vi "SP_BreakDown_Manage1.vi"() -> ()   [LabVIEW 2017]
uses:
  <vilib>/addons/database/Connection.llb/DB Tools Open Connec (Path).vi
  Globle/Login Data.vi
  <vilib>/addons/database/NI_Database_API.lvlib
panel:
  in  "Cancel Button - Archive":bool
  out "Stakeholder":string
  out "Role Id":string
  in  "Download 2":bool
  in  "Get Rport 2":bool
  in  "Manage 2":bool
  out "Table 2":string[][](array[string])
  out "error out":errorcluster
  in  "error in (no error)":errorcluster
  out "Table":string[][](table)
  in  "Shift":string(combo)
  in  "Station":string(combo)
  in  "To Date":timestamp format="%<%Y-%m-%d>T"
  in  "From Date":timestamp format="%<%Y-%m-%d>T"
  in  "Stakeholder":string(combo)
  # "Breakdown Manage"
  # "Designed And Developed By - Infinity Automation Systems Pvt. Ltd."
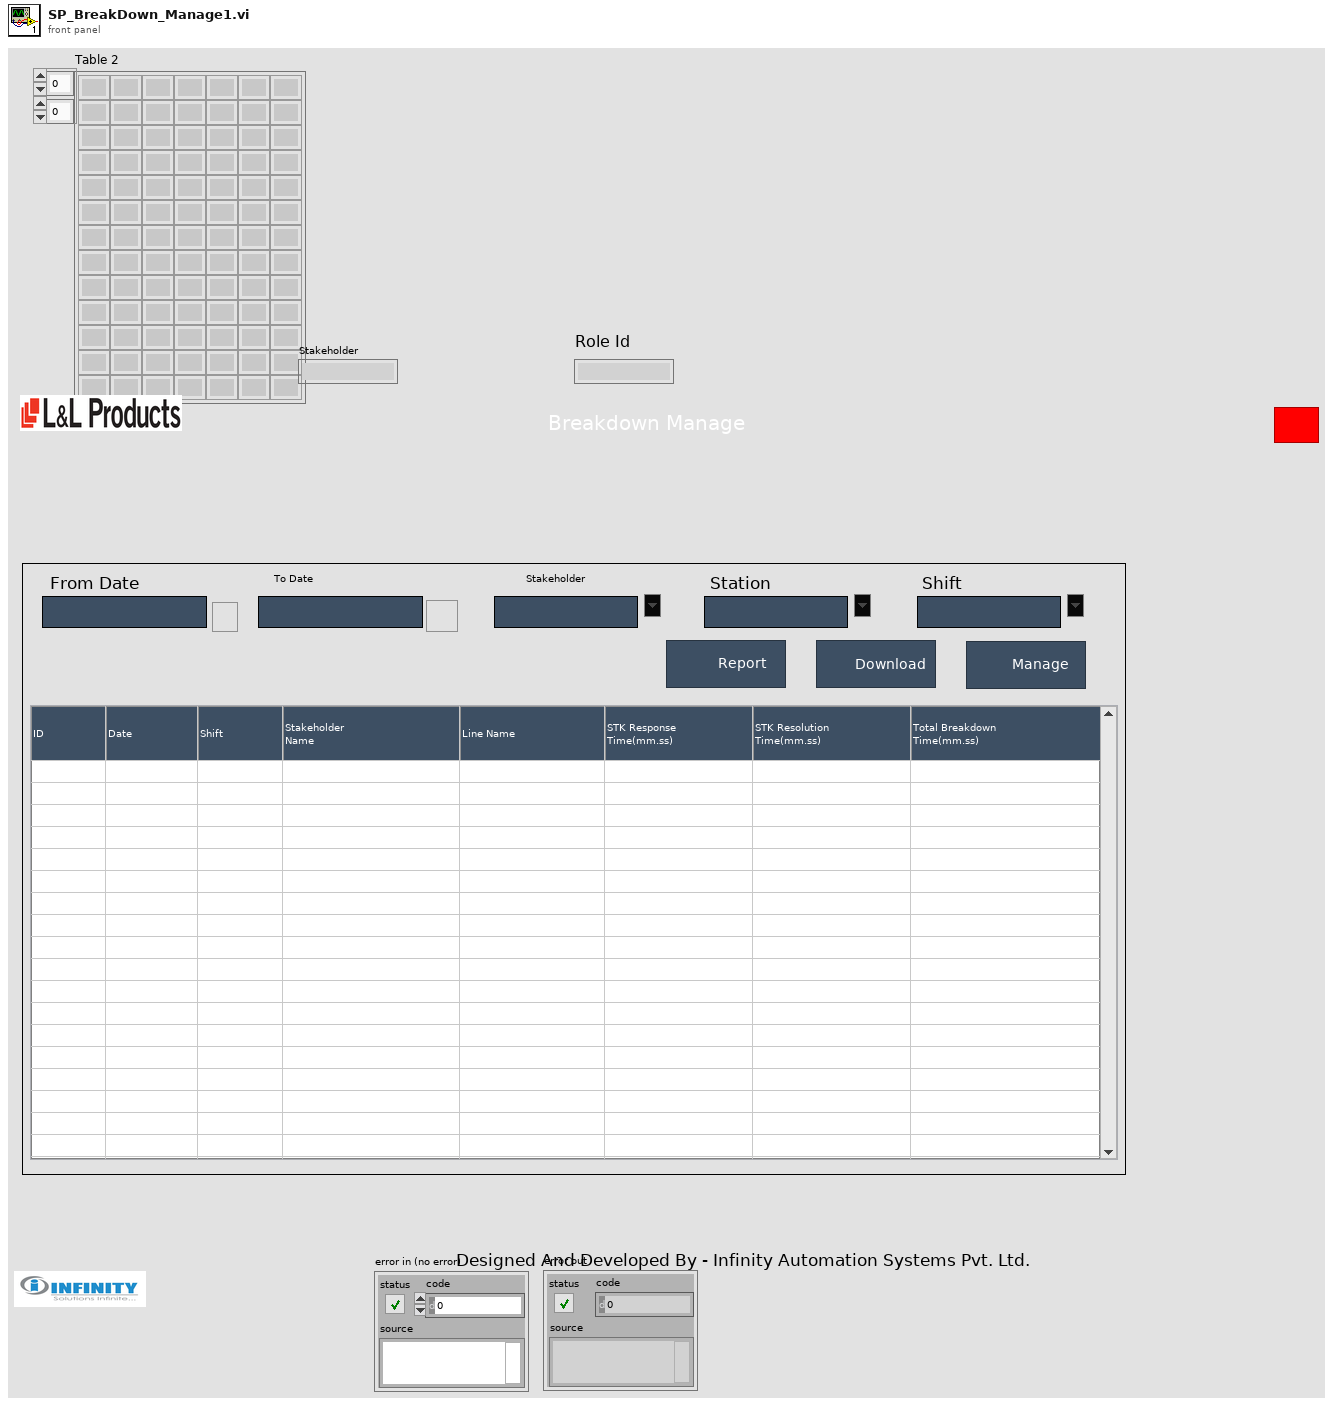
[diagram p1: front panel]
types:
  T1 = typedef "NI_Database_API.lvlib/Conn ObjectReference.ctl" = refnum<k1>
  T2 = enum32{"invalid app kind", "Development System", "Run Time System", "Student Edition", "Embedded LabVIEW", "Evaluation", "Custom"}
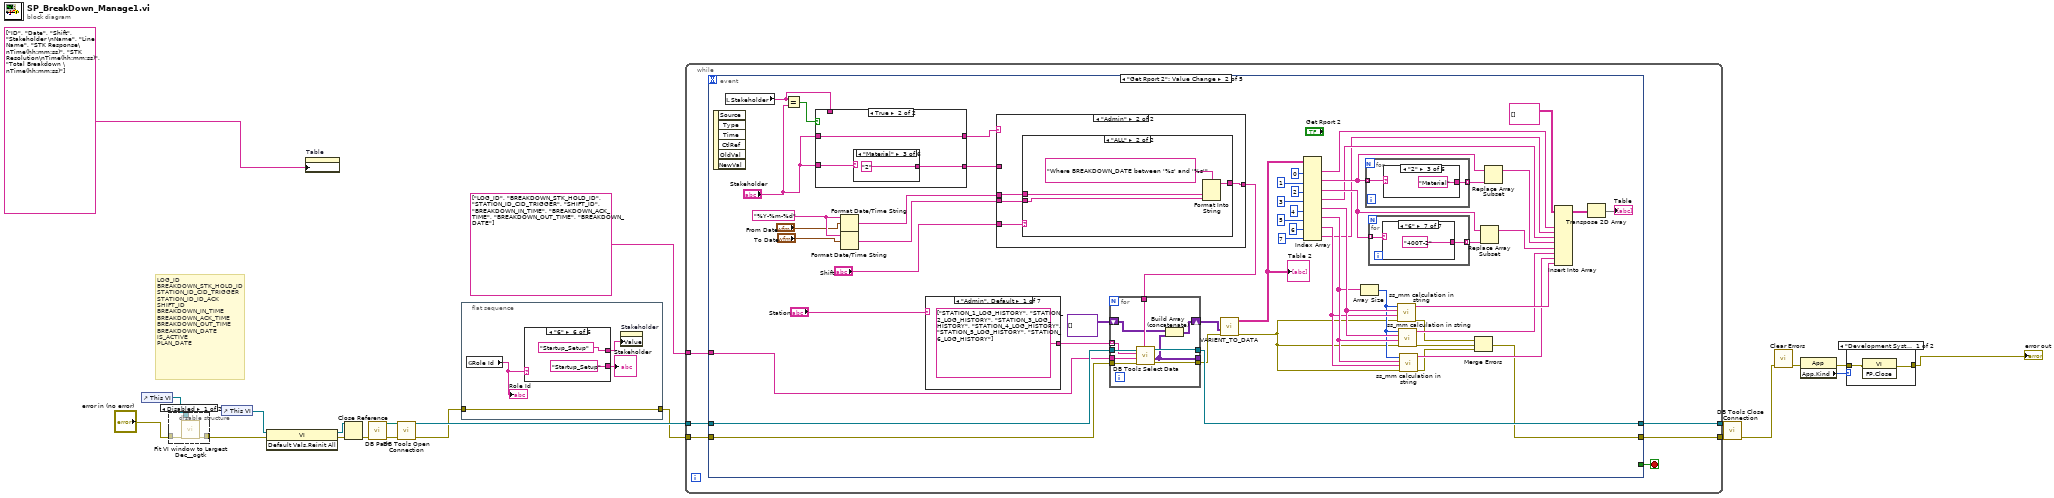
[diagram p0: block diagram]
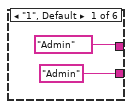
[diagram p3: hidden frame]
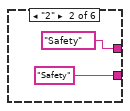
[diagram p4: hidden frame]
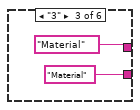
[diagram p5: hidden frame]
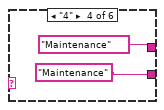
[diagram p6: hidden frame]
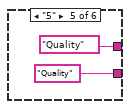
[diagram p7: hidden frame]
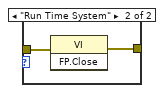
[diagram p8: hidden frame]
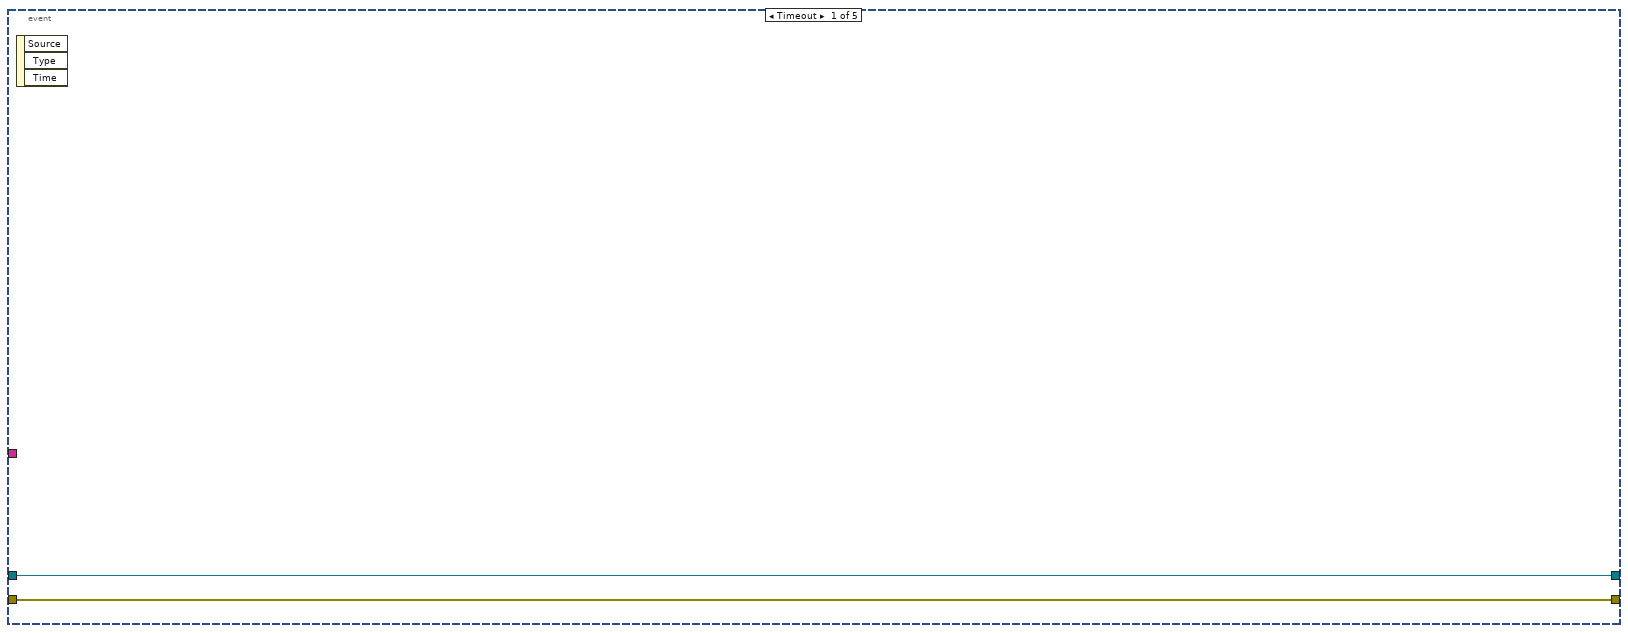
[diagram p9: hidden frame]
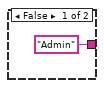
[diagram p10: hidden frame]
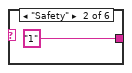
[diagram p12: hidden frame]
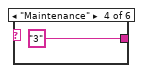
[diagram p13: hidden frame]
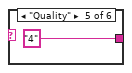
[diagram p14: hidden frame]
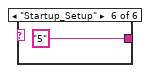
[diagram p15: hidden frame]
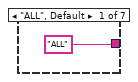
[diagram p16: hidden frame]
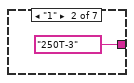
[diagram p17: hidden frame]
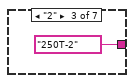
[diagram p18: hidden frame]
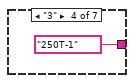
[diagram p19: hidden frame]
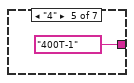
[diagram p20: hidden frame]
diagram:
  # "LOG_ID\nBREAKDOWN_STK_HOLD_ID\nSTATION_ID_CID_TRIGGER\nSTATION_ID_ID_ACK\nSHIFT_ID\nBREAKDOWN_IN_TIME\nBREAKDOWN_ACK_TIME\nBREAKDOWN_OUT_TIME\nBREAKDOWN_DATE\nIS_ACTIVE\nPLAN_DATE"
  n1 = control-ref of="This VI"() -> (w8:refnum<vi>)
  n2 = disable-structure shown="Disabled" {
    disable-tunnel: "error in (no error)" -> [w24 _]
    disable-tunnel: [w23 _] -> w9
    disable-tunnel: w8 -> [w22 _]
    frame Disabled {
      n3 = call <userlib>:"Fit VI window to Largest Dec__ogtk.vi"("error in (no error)"=w24, "VI Ref (calling VI)"=w22) -> ("error out"=w23:errorcluster)  [unwired: 4 in, 1 out]
    }
    frame Enabled {
    }
  }
  n4 = control-ref of="This VI"() -> (w21:refnum<vi>)
  n5 = invoke class="VI" method="Default Vals.Reinit All"(reference=w21, error in=w9) -> (reference out=w19:refnum<vi>, error out=w20:errorcluster)  [unwired: 1 in, 1 out]
  n6 = property on="Table" class="Tbl (strict)"("Column Headers[]"=string[] ["ID", "Date", "Shift", "Stakeholder \nName", "Line Name", "STK Response\nTime(hh:mm:ss)", "STK Resolution\nTime(hh:mm:ss)", "Total Breakdown \nTime(hh:mm:ss)"] ("Column Header Strings[]")) -> ()  [unwired: 2 in, 2 out]
  n7 = Close Reference(reference=w19, error in (no error)=w20) -> (error out=w18:errorcluster)
  n8 = call "DB Path.vi"("error in"=w18) -> ("error out"=w17:errorcluster, "DB Path"=w16:path)  [unwired: 9 in]
  n9 = call-poly <vilib>:"DB Tools Open Connection.vi"("error in (no error)"=w17, "connection information"=w16) -> ("error out"=w2:errorcluster, "connection reference"=w15:T1)  [unwired: 6 in]
  n10 = flat-sequence {
    tunnel: [w28] -> w1
    tunnel: w2 -> [w28]
    frame #0 {
      n11 = global read "Login Data.vi" "Role Id"() -> (w25:string)
      "Role Id" <- w25
      n12 = case shown="\"6\"" w25 {
        tunnel: ["Admin" ("string") "Safety" "Material" "Maintenance" "Quality" "Startup_Setup"] -> w26
        tunnel: ["Admin" ("Stakeholder") "Safety" ("Stakeholder") "Material" ("Stakeholder") "Maintenance" ("Stakeholder") "Quality" ("Stakeholder") "Startup_Setup" ("Stakeholder")] -> w27
        frame "1", Default {
        }
        frame "2" {
        }
        frame "3" {
        }
        frame "4" {
        }
        frame "5" {
        }
        frame "6" {
        }
      }
      "Stakeholder" <- w26
      n13 = property on="Stakeholder" class="CmbBox"("Value"=w27) -> ()  [unwired: 2 in, 2 out]
    }
  }
  n14 = while {
    tunnel: w15 -> [w46]
    tunnel: w1 -> [w45]
    tunnel: [w44] -> w14
    tunnel: [w43] -> w13
    tunnel: string[] ["LOG_ID", "BREAKDOWN_STK_HOLD_ID", "STATION_ID_CID_TRIGGER", "SHIFT_ID", "BREAKDOWN_IN_TIME", "BREAKDOWN_ACK_TIME", "BREAKDOWN_OUT_TIME", "BREAKDOWN_DATE"] -> [w42]
    stop <- w41 stop-if-true
    n15 = event shown="[1] \"Get Rport 2\": Value Change" {
      selector: _ -> [_ _ _ _ _]
      dyn-events: _ -> [_ _ _ _ _]
      timeout: _ -> [_ _ _ _ _]
      tunnel: w46 -> [w47 w93 w177 w180 w184]
      tunnel: w45 -> [w48 w91 w179 w182 w185]
      tunnel: [w48 w55 w178 w181 w185] -> w44
      tunnel: [w47 w92 w177 w180 w184] -> w43
      tunnel: w42 -> [_ w88 _ _ _]
      tunnel: [_ _ _ _ "Cancel Button - Archive"] -> w41
      event Timeout {
        n16 = event-data() -> ()  [unwired: 1 in, 3 out]
      }
      event "Get Rport 2": Value Change {
        w102 = "%Y-%m-%d" ("time format string (%c)")
        n17 = event-data() -> ()  [unwired: 1 in, 6 out]
        n18 = local read "Stakeholder"() -> (w51:string)
        n19 = Equal?(x=w51, y="Stakeholder") -> (x = y?=w52:bool)
        n20 = case shown="True" w52 {
          tunnel: "Stakeholder" -> [_ w105]
          tunnel: [_ w104] -> w96
          tunnel: w51 -> [_ _]
          tunnel: ["Admin" ("Stakeholder") w106] -> w50
          tunnel: "Stakeholder" -> [_ w106]
          frame False {
          }
          frame True {
            n21 = case shown="\"Material\"" w105 {
              tunnel: [_ "1" "2" "3" "4" "5"] -> w104
              frame "Admin", Default {
              }
              frame "Safety" {
              }
              frame "Material" {
              }
              frame "Maintenance" {
              }
              frame "Quality" {
              }
              frame "Startup_Setup" {
              }
            }
          }
        }
        n22 = Format Date/Time String(time format string (%c)=w102, seconds (now)="From Date") -> (date/time string=w98:string)  [unwired: 1 in]
        n23 = Format Date/Time String(time format string (%c)=w102, seconds (now)="To Date") -> (date/time string=w97:string)  [unwired: 1 in]
        n24 = case shown="\"Admin\", Default" "Station" {
          tunnel: [string[] ["STATION_1_LOG_HISTORY", "STATION_2_LOG_HISTORY", "STATION_3_LOG_HISTORY", "STATION_4_LOG_HISTORY", "STATION_5_LOG_HISTORY", "STATION_6_LOG_HISTORY"] string[] ["STATION_1_LOG_HISTORY"] string[] ["STATION_2_LOG_HISTORY"] string[] ["STATION_3_LOG_HISTORY"] string[] ["STATION_4_LOG_HISTORY"] string[] ["STATION_5_LOG_HISTORY"] string[] ["STATION_6_LOG_HISTORY"]] -> w90
          frame "Admin", Default {
          }
          frame "ST 1" {
          }
          frame "ST 2" {
          }
          frame "ST 3" {
          }
          frame "ST 4" {
          }
          frame "ST 5" {
          }
          frame "ST 6" {
          }
        }
        n25 = case shown="\"Admin\"" w50 {
          tunnel: [w149 w165] -> w95
          tunnel: "Shift" -> [w150 w164]
          tunnel: w98 -> [w148 w163]
          tunnel: w97 -> [w147 w162]
          tunnel: w96 -> [w146 _]
          frame "False", Default {
            n26 = case shown="\"ALL\"" w150 {
              selector: w150 -> [w151 _]
              tunnel: [w155 w160] -> w149
              tunnel: w148 -> [w154 w159]
              tunnel: w147 -> [w153 w158]
              tunnel: w146 -> [w152 w157]
              frame "False", Default {
                n27 = Format Into String(format string="Where BREAKDOWN_DATE between '%s' and '%s' and BREAKDOWN_STK_HOLD_ID ='%s'  and SHIFT_ID='%s'  " ("condition"), w154, w153, w152, w151) -> (resulting string=w155:string)  [unwired: 2 in, 1 out]
              }
              frame "ALL" {
                n28 = Format Into String(format string="Where BREAKDOWN_DATE between '%s' and '%s' and BREAKDOWN_STK_HOLD_ID = '%s' " ("condition"), w159, w158, w157) -> (resulting string=w160:string)  [unwired: 2 in, 1 out]
              }
            }
          }
          frame "Admin" {
            n29 = case shown="\"ALL\"" w164 {
              selector: w164 -> [w166 _]
              tunnel: [w169 w173] -> w165
              tunnel: w163 -> [w168 w172]
              tunnel: w162 -> [w167 w171]
              frame "False", Default {
                n30 = Format Into String(format string="Where BREAKDOWN_DATE between '%s' and '%s' and SHIFT_ID='%s'  " ("condition"), w168, w167, w166) -> (resulting string=w169:string)  [unwired: 2 in, 1 out]
              }
              frame "ALL" {
                n31 = Format Into String(format string="Where BREAKDOWN_DATE between '%s' and '%s'" ("condition"), w172, w171) -> (resulting string=w173:string)  [unwired: 2 in, 1 out]
              }
            }
          }
        }
        n32 = for {
          tunnel: w90 -> [w143] mode=indexing
          tunnel: [w137] -> _
          tunnel: w88 -> [w139]
          tunnel: w95 -> [w140]
          tunnel: w91 -> [w142]
          tunnel: [w141] -> w86
          tunnel: w93 -> [w145]
          tunnel: [w144] -> w92
          shift-right: [w136] -> w87
          shift-left: variant[][] [] ("data") -> [w138]
          n33 = call <vilib>:"DB Tools Select Data.vi"("condition"=w140, "error in (no error)"=w142, "columns"=w139, "table"=w143, "connection reference"=w145) -> ("error out"=w141:errorcluster, "data"=w137:variant[][], "connection reference out"=w144:T1)  [unwired: 1 in]
          n34 = Build Array (concatenate)(w138, w137) -> (w136:variant[][])
        }
        n35 = call "VARIENT_TO_DATA.vi"("data"=w87, "error in (no error)"=w86) -> ("Table"=w85:string[][], "error out"=w59:errorcluster)  [unwired: 7 in]
        "Table 2" <- w85
        n36 = Index Array(array=w85, index (col) #1=0 ("disabled index (col)"), index (col) #2=1 ("disabled index (col)"), index (col) #3=2 ("disabled index (col)"), index (col) #4=3 ("disabled index (col)"), index (col) #5=4 ("disabled index (col)"), index (col) #6=5 ("disabled index (col)"), index (col) #7=6 ("disabled index (col)"), index (col) #8=7 ("disabled index (col)")) -> (element #1=w72:string[], element #2=w81:string[], element #3=w79:string[], element #4=w70:string[], element #5=w66:string[], element #6=w65:string[], element #7=w64:string[], element #8=w53:string[])  [unwired: 8 in]
        n37 = Array Size(array=w65) -> (size(s)=w60:i32)
        n38 = for {
          tunnel: w81 -> [w122] mode=indexing
          tunnel: [w121] -> w82 mode=indexing
          n39 = case shown="\"2\"" w122 {
            tunnel: ["all" "Safety" "Material" "Maintenance" "Quality" "Startup_Setup"] -> w121
            frame "False", Default {
            }
            frame "1" {
            }
            frame "2" {
            }
            frame "3" {
            }
            frame "4" {
            }
            frame "5" {
            }
          }
        }
        n40 = for {
          tunnel: w79 -> [w113] mode=indexing
          tunnel: [w112] -> w78 mode=indexing
          n41 = case shown="\"6\"" w113 {
            tunnel: ["ALL" "250T-3" "250T-2" "250T-1" "400T-1" "150T-1" "400T-2"] -> w112
            frame "ALL", Default {
            }
            frame "1" {
            }
            frame "2" {
            }
            frame "3" {
            }
            frame "4" {
            }
            frame "5" {
            }
            frame "6" {
            }
          }
        }
        n42 = call "ss_mm calculation in string.vi"("error in (no error)"=w59, "Table 2"=w64, "Table"=w66, "Numeric"=w60) -> ("error out"=w58:errorcluster, "Array 2"=w63:string[])  [unwired: 6 in]
        n43 = call "ss_mm calculation in string.vi"("error in (no error)"=w59, "Table 2"=w65, "Table"=w66, "Numeric"=w60) -> ("error out"=w57:errorcluster, "Array 2"=w62:string[])  [unwired: 6 in]
        n44 = call "ss_mm calculation in string.vi"("error in (no error)"=w59, "Table 2"=w64, "Table"=w65, "Numeric"=w60) -> ("error out"=w56:errorcluster, "Array 2"=w61:string[])  [unwired: 6 in]
        n45 = Merge Errors(w58, w57, w56) -> (w55:errorcluster)
        n46 = Replace Array Subset(array=w79, new element=w78) -> (w69:string[])  [unwired: 1 in]
        n47 = Replace Array Subset(array=w81, new element=w82) -> (w71:string[])  [unwired: 1 in]
        n48 = Insert Into Array(array=string[][] [], new element #1=w72, new element #2=w53, new element #3=w70, new element #4=w71, new element #5=w69, new element #6=w62, new element #7=w61, new element #8=w63) -> (w68:string[][])  [unwired: 2 in]
        n49 = Transpose 2D Array(2D array=w68) -> (transposed array=→"Table":string[][])
      }
      event "Download 2": Value Change {
        n50 = event-data() -> ()  [unwired: 1 in, 6 out]
        n51 = local read "Table"() -> (w175:string[][])
        n52 = call "Download_Report_subvi.vi"("error in (no error)"=w179, "Value"=w175, "Column Header Strings[]"=string[][] [["ID", "Date", "Shift", "Stakeholder \nName", "Line Name", "STK Response\nTime(mm.ss)", "STK Resolution\nTime(mm.ss)", "Total Breakdown \nTime(mm.ss)"]]) -> ("error out"=w178:errorcluster)  [unwired: 8 in]
      }
      event "Manage 2": Value Change {
        n53 = event-data() -> ()  [unwired: 1 in, 6 out]
        n54 = call "manage breakdown sub.vi"("error in (no error)"=w182) -> ("error out"=w181:errorcluster)  [unwired: 10 in]
      }
      event "Cancel Button - Archive": Value Change {
        n55 = event-data() -> ()  [unwired: 1 in, 6 out]
      }
    }
  }
  n56 = call <vilib>:"DB Tools Close Connection.vi"("error in (no error)"=w14, "connection reference"=w13) -> ("error out"=w4:errorcluster)  [unwired: 5 in]
  n57 = call <vilib>:"Clear Errors.vi"("error in (no error)"=w4) -> ("error out"=w7:errorcluster)  [unwired: 5 in, 1 out]
  n58 = property class="App"(error in=w7) -> (error out=w6:errorcluster, "App.Kind"=w5:T2)  [unwired: 1 in, 1 out]
  n59 = case shown="\"Development System\", Default" w5 {
    tunnel: w6 -> [w187 w189]
    tunnel: [w186 w188] -> w3
    frame "Development System", Default {
      n60 = invoke class="VI" method="FP.Close"(error in=w187) -> (error out=w186:errorcluster)  [unwired: 2 in, 2 out]
    }
    frame "Run Time System" {
      n61 = invoke class="VI" method="FP.Close"(error in=w189) -> (error out=w188:errorcluster)  [unwired: 2 in, 2 out]
    }
  }
  "error out" <- w3
